vi "SPI Read Data.vi"(7 "SPI #":T1=-1, 8 "error in (no error)":errorcluster, 9 "Len":u8, 11 "VisaComms in":refnum<class "VisaComms.lvclass">) -> (0 "error out":errorcluster, 1 "Data":string, 3 "VisaComms out":refnum<class "VisaComms.lvclass">)   [LabVIEW 2020, in "CTI.lvlib" / "VisaComms.lvclass"]
uses:
  VisaComms.lvclass
  SPI Number.ctl
  VisaComms.lvclass/VisaComms.ctl
  Clean Visa Errors.vi
  CTI.lvlib
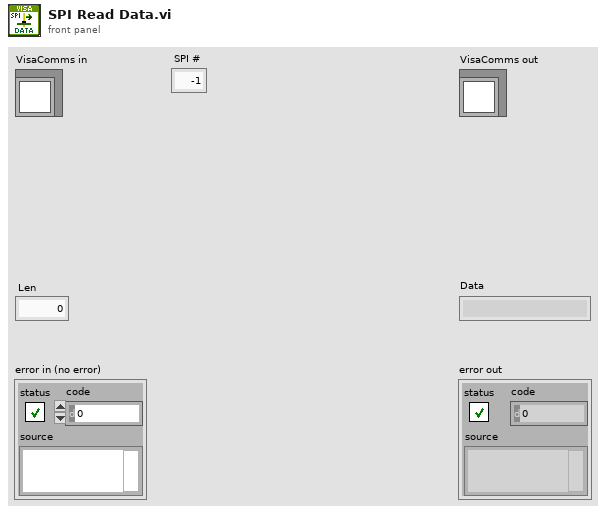
[diagram p1: front panel]
types:
  T1 = typedef "CTI.lvlib/SPI Number.ctl" = i8
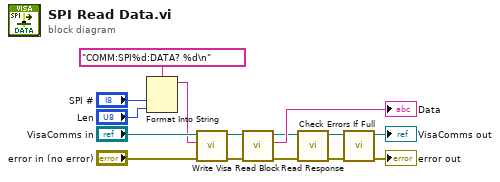
[diagram p0: block diagram]
diagram:
  n1 = Format Into String(format string="COMM:SPI%d:DATA? %d\n", "SPI #", "Len") -> (resulting string=w9:string)  [unwired: 2 in, 1 out]
  n2 = call "Write Visa.vi"("error in (no error)"="error in (no error)", "write buffer"=w9, "VisaComms in"="VisaComms in") -> ("error out"=w11:errorcluster, "VisaComms out"=w7:refnum<class "VisaComms.lvclass">)  [unwired: 6 in, 1 out]
  n3 = call "Read Block.vi"("error in (no error)"=w11, "VisaComms in"=w7) -> ("error out"=w8:errorcluster, "Block"=→"Data":string, "VisaComms out"=w4:refnum<class "VisaComms.lvclass">)  [unwired: 6 in, 1 out]
  n4 = call "Read Response.vi"("error in (no error)"=w8, "VisaComms in"=w4) -> ("error out"=w5:errorcluster, "VisaComms out"=w2:refnum<class "VisaComms.lvclass">)  [unwired: 6 in, 2 out]
  n5 = call "Check Errors If Full.vi"("error in (no error)"=w5, "VisaComms in"=w2) -> ("error out"=→"error out":errorcluster, "VisaComms out"=→"VisaComms out":refnum<class "VisaComms.lvclass">)  [unwired: 8 in]
